vi "Subscribe.vi"(8 "error in (no error)":errorcluster, 9 "Subscriber Enqueuer":refnum<class "Message Enqueuer.lvclass">, 10 "Topic":string, 11 "Broadcaster in":refnum<class "BroadcastBroker.lvclass">) -> (0 "error out":errorcluster, 3 "Broadcaster out":refnum<class "BroadcastBroker.lvclass">)   [LabVIEW 2019, in "BroadcastBroker.lvclass"]
uses:
  BroadcastBroker.lvclass
  <vilib>/ActorFramework/Message Enqueuer/Message Enqueuer.lvclass
  BroadcastBroker.lvclass/BroadcastBroker.ctl
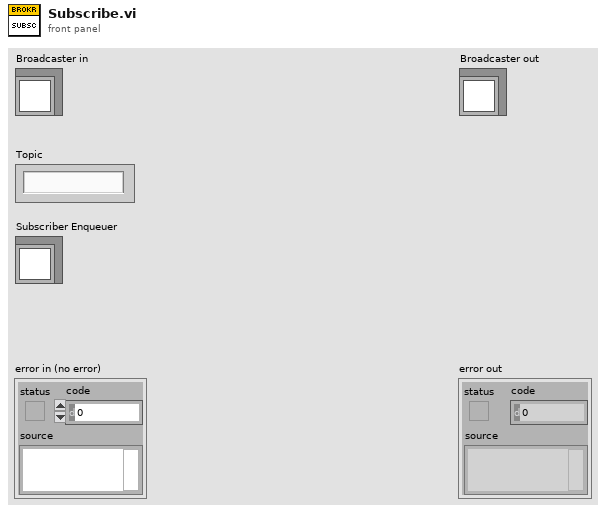
[diagram p1: front panel]
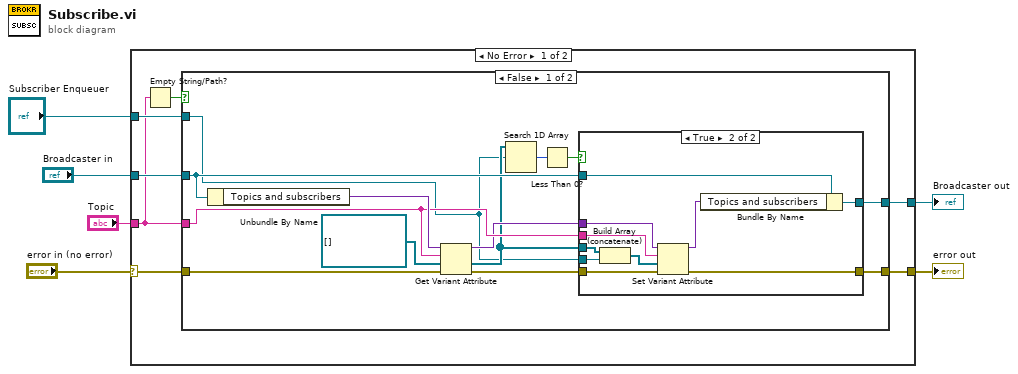
[diagram p0: block diagram]
diagram:
  n1 = case shown="No Error" "error in (no error)" {
    selector: "error in (no error)" -> [w12 w42]
    tunnel: [w10 w42] -> w5
    tunnel: [w11 w41] -> w3
    tunnel: "Broadcaster in" -> [w13 w41]
    tunnel: "Topic" -> [w8 _]
    tunnel: "Subscriber Enqueuer" -> [w9 _]
    frame No Error {
      n2 = Empty String/Path?(string/path=w8) -> (empty?=w7:bool)
      n3 = case shown="False" w7 {
        tunnel: w13 -> [w26 w40]
        tunnel: w12 -> [w24 w39]
        tunnel: w8 -> [w22 _]
        tunnel: [w19 w40] -> w11
        tunnel: [w18 w39] -> w10
        tunnel: w9 -> [w16 _]
        frame False {
          n4 = Unbundle By Name(w26) -> ("Topics and subscribers"=w25:variant)
          n5 = Get Variant Attribute(Variant=w25, name=w22, default value (empty Variant)=refnum<class "Message Enqueuer.lvclass">[] [], error in=w24) -> (duplicate Variant=w20:variant, value=w17:refnum<class "Message Enqueuer.lvclass">[], error out=w21:errorcluster)  [unwired: 1 out]
          n6 = Search 1D Array(1D array=w17, element=w16) -> (index of element=w15:i32)  [unwired: 1 in]
          n7 = Less Than 0?(x=w15) -> (x < 0?=w14:bool)
          n8 = case shown="True" w14 {
            tunnel: w26 -> [w28 w38]
            tunnel: w22 -> [_ w37]
            tunnel: w21 -> [w27 w36]
            tunnel: w20 -> [_ w34]
            tunnel: [w28 w33] -> w19
            tunnel: [w27 w31] -> w18
            tunnel: w17 -> [_ w30]
            tunnel: w16 -> [_ w29]
            frame False {
            }
            frame True {
              n9 = Build Array (concatenate)(w30, w29) -> (w35:refnum<class "Message Enqueuer.lvclass">[])
              n10 = Set Variant Attribute(Variant=w34, name=w37, value=w35, error in=w36) -> (Variant out=w32:variant, error out=w31:errorcluster)  [unwired: 1 out]
              n11 = Bundle By Name(cluster=w38, "Topics and subscribers"=w32) -> (w33:refnum<class "BroadcastBroker.lvclass">)
            }
          }
        }
        frame True {
        }
      }
    }
    frame Error {
    }
  }
  "error out" <- w5
  "Broadcaster out" <- w3
